vi "SP Find Filter Limit by Parameter.vi"(9 "Display Format":T1=7 items=["Log Mag", "Phase", "Expanded Phase", "Delay", "Smith", "Polar", "Lin Mag", "SWR", "Loss", "Real", "Imaginary"], 10 "Parameter":T2={"Stimulus Port"=1, "Response Port"=1} caption="Parameter String" {"Stimulus Port" min=1 step=1; "Response Port" min=1 step=1}, 11 "Filter Limits":T3[](array[typedef]) {"Parameter"."Stimulus Port" min=1 step=1; "Parameter"."Response Port" min=1 step=1; "Passband"."Bandwidth Attn" format="%.3g"; "Passband"."Stop/Span" format="%.3g"; "Passband"."Start/Center" format="%.3g"}) -> (0 "Found?":bool, 3 "Filter Limits":T3[](array[typedef]) {"Parameter"."Stimulus Port" min=1 step=1; "Parameter"."Response Port" min=1 step=1; "Passband"."Bandwidth Attn" format="%.3g"; "Passband"."Stop/Span" format="%.3g"; "Passband"."Start/Center" format="%.3g"})   [LabVIEW 2011]
uses:
  TypeDefs/SP Filter.ctl
  TypeDefs/SP Parameter.ctl
  TypeDefs/SP Format.ctl
  TypeDefs/SP Filter Type.ctl
  TypeDefs/SP Filter Passband.ctl
  TypeDefs/SP Frequency Units.ctl
  TypeDefs/SP Frequency Format.ctl
  TypeDefs/SP Filter Ripple.ctl
  TypeDefs/SP Attenuation Point.ctl
  TypeDefs/SP Attenuation Type.ctl
  TypeDefs/SP Skirt Rejection Point.ctl
  TypeDefs/SP Relative Loss.ctl
  TypeDefs/SP Display Format.ctl
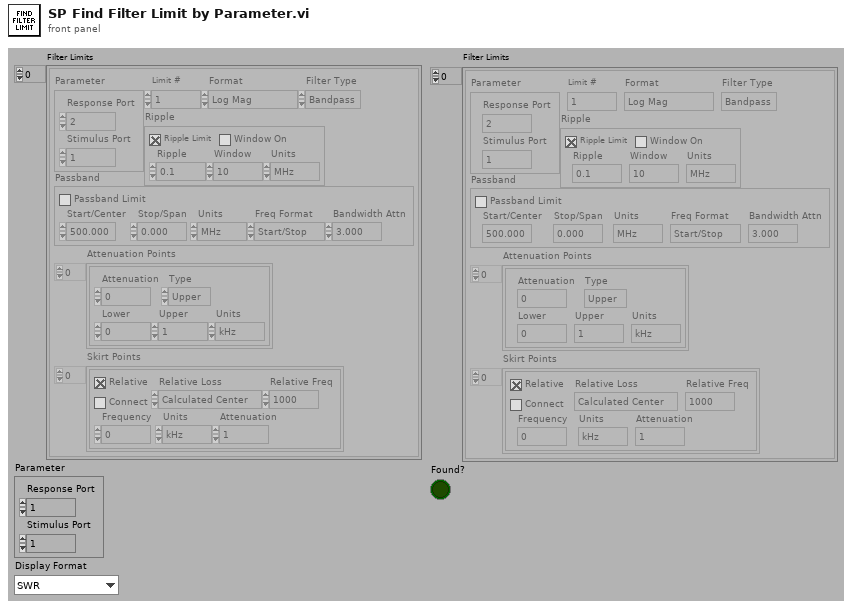
[diagram p1: front panel]
types:
  T1 = typedef "SP Display Format.ctl" = i32
  T2 = typedef "SP Parameter.ctl" = cluster{"Stimulus Port":i8, "Response Port":i8}
  T3 = typedef "SP Filter.ctl" = cluster{"Limit #":i8, "Parameter":T2, "Format":T4, "Filter Type":T5, "Passband":T6, "Ripple":T9, "Attenuation Points":T10[], "Skirt Points":T12[]}
  T4 = typedef "SP Format.ctl" = enum16{"Log Mag", "Lin Mag", "SWR", "Phase", "Expanded Phase", "Delay", "Insertion Loss", "Isolation", "Return Loss"}
  T5 = typedef "SP Filter Type.ctl" = enum16{"Lowpass", "Highpass", "Bandpass", "Bandstop"}
  T6 = typedef "SP Filter Passband.ctl" = cluster{"Start/Center":dbl, "Stop/Span":dbl, "Units":T7, "Freq Format":T8, "Bandwidth Attn":dbl, "Passband Limit":bool}
  T7 = typedef "SP Frequency Units.ctl" = enum16{"Hz", "kHz", "MHz", "GHz", "Points"}
  T8 = typedef "SP Frequency Format.ctl" = enum16{"Start/Stop", "Center/Span"}
  T9 = typedef "SP Filter Ripple.ctl" = cluster{"Ripple Limit":bool, "Window On":bool, "Ripple":dbl, "Window":dbl, "Units":T7}
  T10 = typedef "SP Attenuation Point.ctl" = cluster{"Attenuation":dbl, "Type":T11, "Lower":dbl, "Upper":dbl, "Units":T7}
  T11 = typedef "SP Attenuation Type.ctl" = enum16{"Center", "Lower", "Upper"}
  T12 = typedef "SP Skirt Rejection Point.ctl" = cluster{"Relative":bool, "Connect":bool, "Frequency":dbl, "Units":T7, "Attenuation":dbl, "Relative Loss":T13, "Relative Freq":dbl}
  T13 = typedef "SP Relative Loss.ctl" = enum16{"Calculated Center", "Passband Minimum", "Passband Maximum", "Passband Average", "Frequency"}
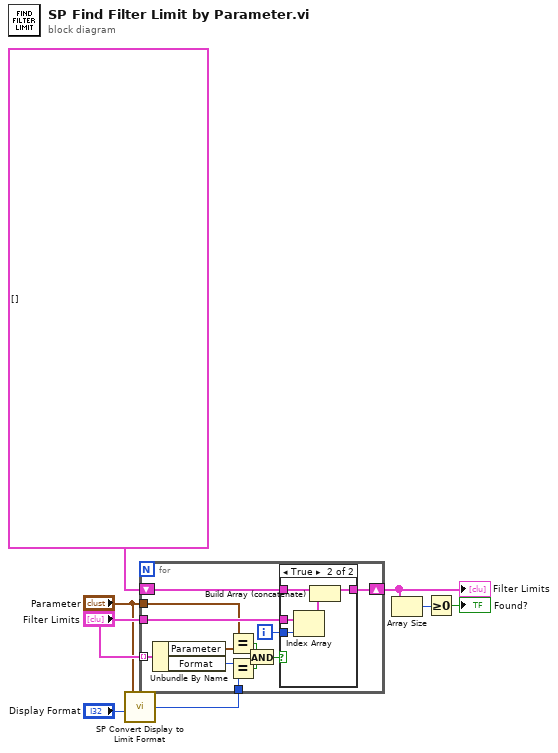
[diagram p0: block diagram]
diagram:
  n1 = call "SP Convert Display to Limit Format.vi"("Display Format"="Display Format", "S Parameter"="Parameter") -> ("Limit Format"=w1:T4)  [unwired: 4 out]
  n2 = for {
    tunnel: "Filter Limits" -> [w20] mode=indexing
    tunnel: "Filter Limits" -> [w19]
    shift-right: [w16] -> w4
    shift-left: T3[] [] ("Limits") -> [w17]
    tunnel: "Parameter" -> [w14]
    tunnel: w1 -> [w11]
    i -> [w18]
    n3 = Unbundle By Name(w20) -> ("Parameter"=w15:T2, "Format"=w12:T4)
    n4 = Equal?(x=w14, y=w15) -> (x = y?=w10:bool)
    n5 = Equal?(x=w12, y=w11) -> (x = y?=w9:bool)
    n6 = And(x=w10, y=w9) -> (x .and. y?=w13:bool)
    n7 = case shown="True" w13 {
      tunnel: w19 -> [_ w26]
      tunnel: w18 -> [_ w25]
      tunnel: w17 -> [w21 w23]
      tunnel: [w21 w22] -> w16
      frame False {
      }
      frame True {
        n8 = Index Array(array=w26, index=w25) -> (element=w24:T3)
        n9 = Build Array (concatenate)(w23, w24) -> (w22:T3[])
      }
    }
  }
  "Filter Limits" <- w4
  n10 = Array Size(array=w4) -> (size(s)=w6:i32)
  n11 = Greater Or Equal To 0?(x=w6) -> (x >= 0?=→"Found?":bool)
